vi "Demo0.vi"   [LabVIEW 2012]
uses:
  <vilib>/NXT/LegoClasses/VIA/VIA.lvclass
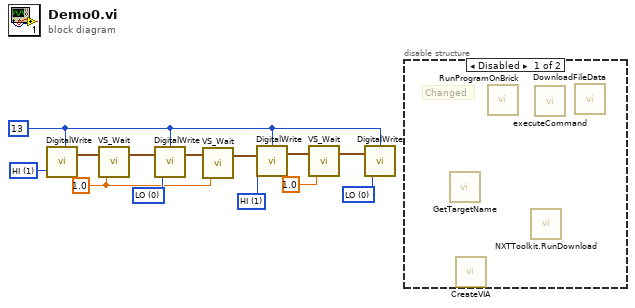
[diagram p0: block diagram]
diagram:
  w8 = u16 0 items=["LO", "HI"] ("State")
  w7 = u16 1 items=["LO", "HI"] ("State")
  w10 = u16 0 items=["LO", "HI"] ("State")
  w11 = u16 1 items=["LO", "HI"] ("State")
  w2 = sgl 1.0 ("delay (s)")
  w1 = u8 13 ("Port")
  n1 = call "DigitalWrite.vi"("State"=w11, "Port"=w1) -> ("Info Out"=w13:cluster{"Numeric":u8})  [unwired: 1 in, 1 out]
  n2 = call "VS_Wait.vi"("delay (s)"=w2, "Info In"=w13) -> ("Info Out"=w12:cluster{"Numeric":u8})  [unwired: 1 in, 1 out]
  n3 = call "DigitalWrite.vi"("State"=w10, "Info In"=w12, "Port"=w1) -> ("Info Out"=w9:cluster{"Numeric":u8})  [unwired: 1 out]
  n4 = call "VS_Wait.vi"("delay (s)"=w2, "Info In"=w9) -> ("Info Out"=w3:cluster{"Numeric":u8})  [unwired: 1 in, 1 out]
  n5 = call "DigitalWrite.vi"("State"=w7, "Info In"=w3, "Port"=w1) -> ("Info Out"=w4:cluster{"Numeric":u8})  [unwired: 1 out]
  n6 = call "VS_Wait.vi"("delay (s)"=sgl 1.0, "Info In"=w4) -> ("Info Out"=w5:cluster{"Numeric":u8})  [unwired: 1 in, 1 out]
  n7 = call "DigitalWrite.vi"("State"=w8, "Info In"=w5, "Port"=w1) -> ()  [unwired: 2 out]
  n8 = disable-structure shown="Disabled" {
    frame Disabled {
      # "Changed"
      n9 = call-dynamic "GetTargetName.vi"() -> ()  [unwired: 9 in, 3 out]
      n10 = call <vilib>:"CreateVIA.vi"() -> ()  [unwired: 11 in, 1 out]
      n11 = call-dynamic "RunProgramOnBrick.vi"() -> ()  [unwired: 10 in, 2 out]
      n12 = call "NXTToolkit.RunDownload.vi"() -> ()  [unwired: 1 in, 1 out]
      n13 = call "executeCommand.vi"() -> ()  [unwired: 6 in, 6 out]
      n14 = call-dynamic "DownloadFileData.vi"() -> ()  [unwired: 8 in, 4 out]
    }
    frame Enabled {
    }
  }
